vi "Yscalingtest.vi"(6 "current":dbl, 8 "Nano Z Read":dbl, 9 "Current Maxed?":bool, 10 "Y":dbl, 11 "Plane Height":dbl) -> (3 "y scaled":dbl, 4 "Testoutput":dbl)   [LabVIEW 2017]
uses:
  HapticSTM.lvlib
panel:
  out "force":T1(graph)
  out "current":cluster{"current":dbl}(graph)
  out "Zpos":T2(graph)
  out "appended array":dbl[](array[numeric])
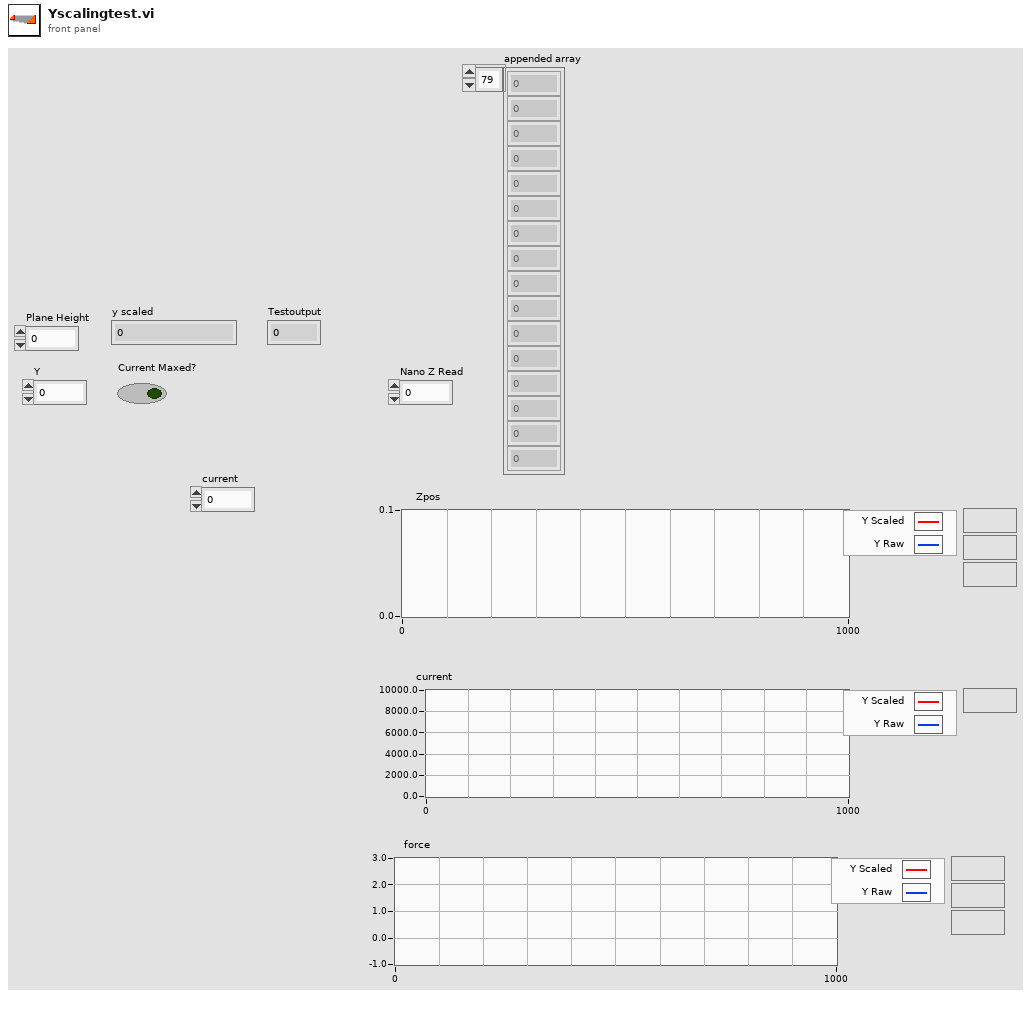
[diagram p1: front panel]
types:
  T1 = cluster{"function return":dbl, "function return":dbl, "function return":dbl}
  T2 = cluster{dbl, "function return":dbl, "function return":dbl}
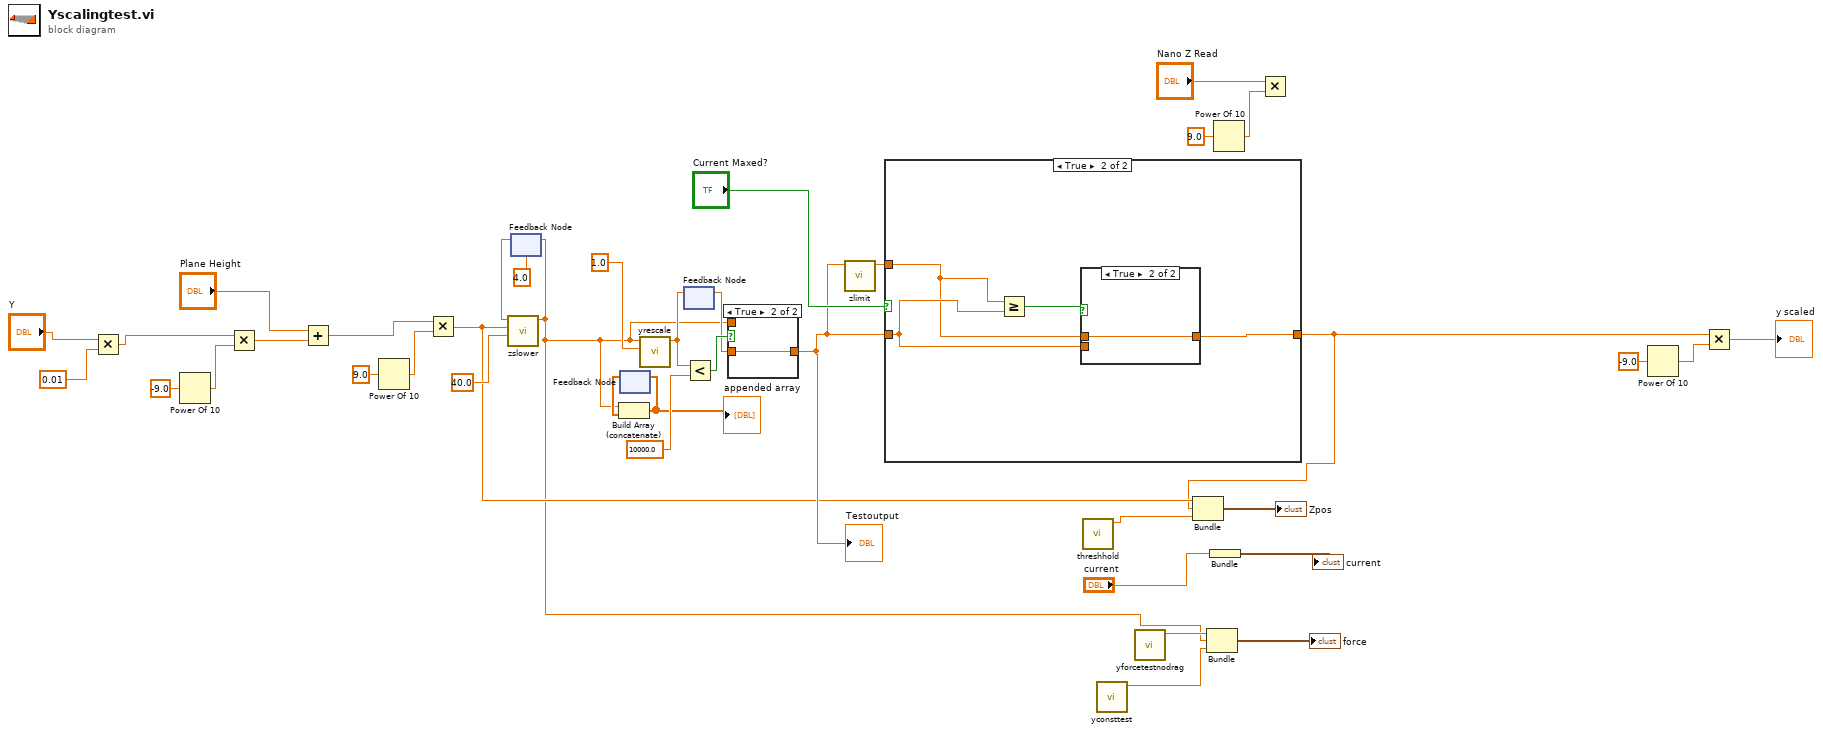
[diagram p0: block diagram]
diagram:
  n1 = Multiply(x="Y", y=0.01) -> (x*y=w35:dbl)
  n2 = Power Of 10(x=-9.0) -> (10^x=w34:dbl)
  n3 = Multiply(x=w35, y=w34) -> (x*y=w36:dbl)
  n4 = Add(x="Plane Height", y=w36) -> (x+y=w39:dbl)
  n5 = Power Of 10(x=9.0) -> (10^x=w38:dbl)
  n6 = Multiply(x=w39, y=w38) -> (x*y=w11:dbl)
  n7 = feedback #1(4.0 ("function return")) -> (w13:dbl)
  n8 = call "zslower.vi"("maxvel"=40.0, "labview_zpos_write"=w11, "nanonis_zpos_read"=w13) -> ("function return"=w2:dbl)  [unwired: 8 in]
  n9 = feedback-in #1(w2) -> ()
  n10 = feedback #2() -> (w15:dbl[])  [unwired: 1 in]
  n11 = Build Array (concatenate)(w2, w15) -> (w16:dbl[])
  "appended array" <- w16
  n12 = feedback-in #2(w16) -> ()
  n13 = call "yrescale.vi"("scalingfactor"=1.0, "ylabview"=w2) -> ("function return"=w3:dbl)  [unwired: 9 in]
  n14 = feedback-in #3(w3) -> ()
  n15 = feedback #3() -> (w20:dbl)  [unwired: 1 in]
  n16 = Less?(x=w3, y=10000.0) -> (x < y?=w21:bool)
  n17 = case shown="True" w21 {
    tunnel: [w40 w41] -> w23
    tunnel: w20 -> [_ w41]
    tunnel: w2 -> [w40 _]
    frame False {
    }
    frame True {
    }
  }
  "Testoutput" <- w23
  n18 = call "zlimit.vi"("yscaledinput"=w23) -> ("function return"=w24:dbl)  [unwired: 10 in]
  n19 = case shown="True" "Current Maxed?" {
    tunnel: [w42 w46] -> w10
    tunnel: w23 -> [w42 w44]
    tunnel: w24 -> [_ w43]
    frame False {
    }
    frame True {
      n20 = Greater Or Equal?(x=w43, y=w44) -> (x >= y?=w45:bool)
      n21 = case shown="True" w45 {
        tunnel: w43 -> [_ w48]
        tunnel: [w47 w48] -> w46
        tunnel: w44 -> [w47 _]
        frame False {
        }
        frame True {
        }
      }
    }
  }
  n22 = call "threshhold.vi"() -> ("function return"=w8:dbl)  [unwired: 11 in]
  n23 = call "yconsttest.vi"() -> ("function return"=w1:dbl)  [unwired: 11 in]
  n24 = call "yforcetestnodrag.vi"() -> ("function return"=w4:dbl)  [unwired: 11 in]
  n25 = Bundle(w11, "function return"=w10, "function return"=w8) -> (→"Zpos":T2)  [unwired: 1 in]
  n26 = Bundle("function return"=w4, "function return"=w2, "function return"=w1) -> (→"force":T1)  [unwired: 1 in]
  n27 = Bundle("current"="current") -> (→"current":cluster{"current":dbl})  [unwired: 1 in]
  n28 = Power Of 10(x=9.0) -> (10^x=w19:dbl)
  n29 = Multiply(x="Nano Z Read", y=w19) -> ()  [unwired: 1 out]
  n30 = Power Of 10(x=-9.0) -> (10^x=w27:dbl)
  n31 = Multiply(x=w10, y=w27) -> (x*y=→"y scaled":dbl)
